vi "2_STAGE.vi"(8 "Dataflow In":errorcluster) -> (0 "Dataflow Out":errorcluster)   [LabVIEW 2019]
panel:
  # "*******************************************************************\nBiogas Plant Control\n\nAuthor: Paul Zügel\nGCSC-Frankfurt am Main 2020\n\n*******************************************************************"
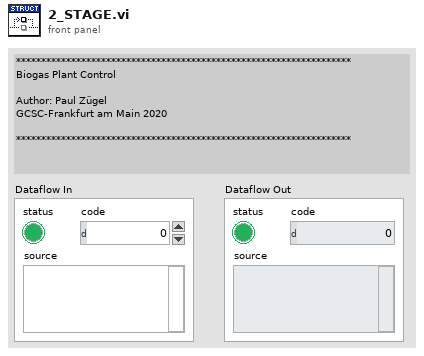
[diagram p1: front panel]
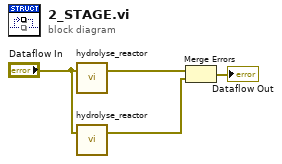
[diagram p0: block diagram]
diagram:
  n1 = call "hydrolyse_reactor.vi"("Dataflow In"="Dataflow In") -> ("Dataflow Out"=w3:errorcluster)  [unwired: 2 in]
  n2 = call "hydrolyse_reactor.vi"("Dataflow In"="Dataflow In") -> ("Dataflow Out"=w2:errorcluster)  [unwired: 2 in]
  n3 = Merge Errors(w3, w2) -> (→"Dataflow Out":errorcluster)
